vi "HW_GEN - Update Units List.vi"(10 "Units[]":string[](array[string]), 11 "Chan dflt Para in":T3) -> (2 "Units out":string, 3 "Chan dflt Para out":T3)   [LabVIEW 2016]
uses:
  Ctrls/HardWare _ Channel Configurations PopUp Type.ctl
  ToolKit/Popup/Private/Ctrls/POP_Data Type.ctl
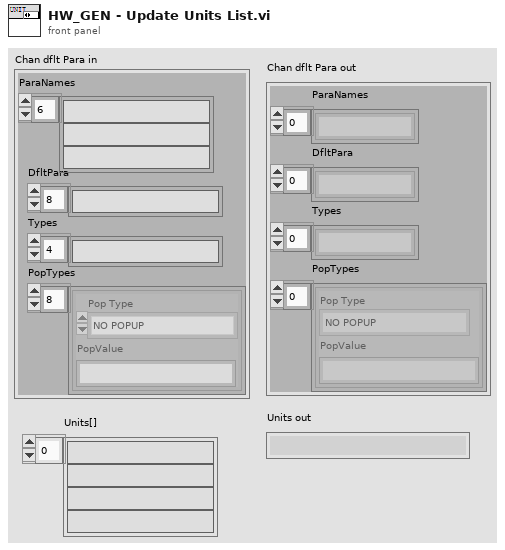
[diagram p1: front panel]
types:
  T1 = typedef "HardWare _ Channel Configurations PopUp Type.ctl" = cluster{"Pop Type":T2, "PopValue":string}
  T2 = typedef "POP_Data Type.ctl" = enum16{"NO POPUP", "Unkown", "String", "Integer", "Float", "Color", "Boolean", "Ring", "Captioned String", "Captioned Integer", "Button Color", "2 Int Cluster", "4 Int Cluster", "6-Dbl Cluster", "Path", "Combox", "Time", "ShotCut String"}
  T3 = cluster{"ParaNames":string[], "DfltPara":string[], "Types":string[], "PopTypes":T1[]}
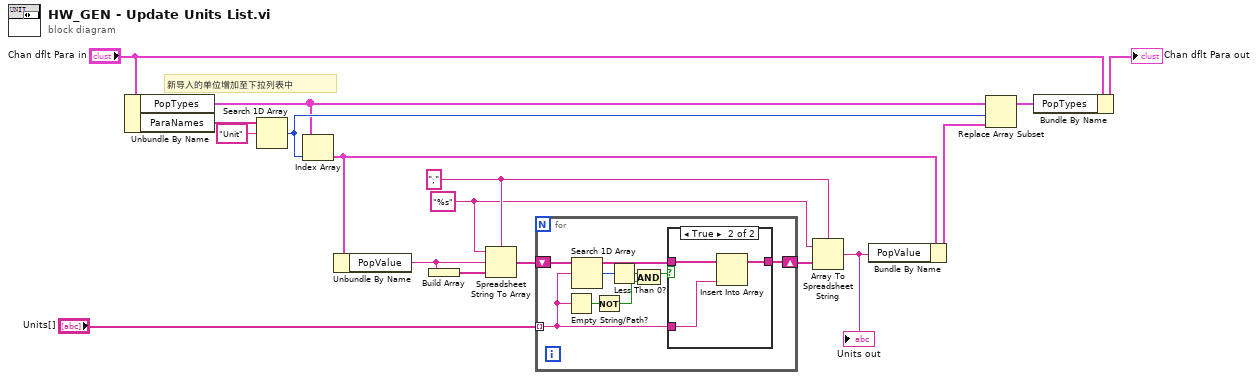
[diagram p0: block diagram]
diagram:
  w7 = "%s" ("format string")
  w9 = "," ("delimiter (Tab)")
  # "新导入的单位增加至下拉列表中"
  n1 = Unbundle By Name("Chan dflt Para in") -> ("PopTypes"=w4:T1[], "ParaNames"=w17:string[])
  n2 = Search 1D Array(1D array=w17, element="Unit") -> (index of element=w6:i32)  [unwired: 1 in]
  n3 = Index Array(array=w4, index=w6) -> (element=w11:T1)
  n4 = Unbundle By Name(w11) -> ("PopValue"=w14:string)
  n5 = Build Array(w14) -> (w15:string[])
  n6 = Spreadsheet String To Array(delimiter (Tab)=w9, format string=w7, spreadsheet string=w14, array type (2D Dbl)=w15) -> (array=w13:string[])
  n7 = for {
    tunnel: "Units[]" -> [w20] mode=indexing
    shift-right: [w23] -> w8
    shift-left: w13 -> [w24]
    n8 = Empty String/Path?(string/path=w20) -> (empty?=w19:bool)
    n9 = Search 1D Array(1D array=w24, element=w20) -> (index of element=w25:i32)  [unwired: 1 in]
    n10 = Not(x=w19) -> (.not. x?=w18:bool)
    n11 = Less Than 0?(x=w25) -> (x < 0?=w22:bool)
    n12 = And(x=w22, y=w18) -> (x .and. y?=w21:bool)
    n13 = case shown="True" w21 {
      tunnel: w24 -> [w26 w29]
      tunnel: w20 -> [_ w28]
      tunnel: [w26 w27] -> w23
      frame False {
      }
      frame True {
        n14 = Insert Into Array(array=w29, new element=w28) -> (w27:string[])  [unwired: 1 in]
      }
    }
  }
  n15 = Array To Spreadsheet String(delimiter (Tab)=w9, array=w8, 3:w7) -> (spreadsheet string=w10:string)
  "Units out" <- w10
  n16 = Bundle By Name(cluster=w11, "PopValue"=w10) -> (w5:T1)
  n17 = Replace Array Subset(array=w4, new element=w5, index=w6) -> (w2:T1[])
  n18 = Bundle By Name(cluster="Chan dflt Para in", "PopTypes"=w2) -> (→"Chan dflt Para out":T3)
